vi "ConfigureFPGATach.vi"(8 "error in (no error)":errorcluster, 9 "delay comp":u32, 10 "keyphasor config":T1[](array[typedef]), 11 "dynamic FPGA VI reference":refnum<k20>) -> (0 "error out":errorcluster, 3 "dynamic FPGA VI reference":refnum<k20>)   [LabVIEW 2017, in "cRIOWfmLib.lvlib"]
uses:
  <vilib>/addons/InsightCM/Devices/Shared/Cms/cRIOWfmAcq/cRIOWfmLib.lvlib
  <vilib>/addons/InsightCM/Devices/Shared/Cms/CmsAcquisition/controls/TachometerConfig.ctl
  <vilib>/Utility/error.llb/Error Cluster From Error Code.vi
  <vilib>/rvi/errors/niLvFpgaAdjustHostInterfaceError.vi
  <vilib>/rvi/interface/nirviReadWriteControl/nirviReadWriteControl.xnode
  NiFpgaLv.dll
  <vilib>/rvi/interface/Simulation/niFpgaSimulationCallBeginRW.vi
  <vilib>/addons/InsightCM/Devices/Shared/Cms/CmsAcquisition/CmsAcquisition.lvlib
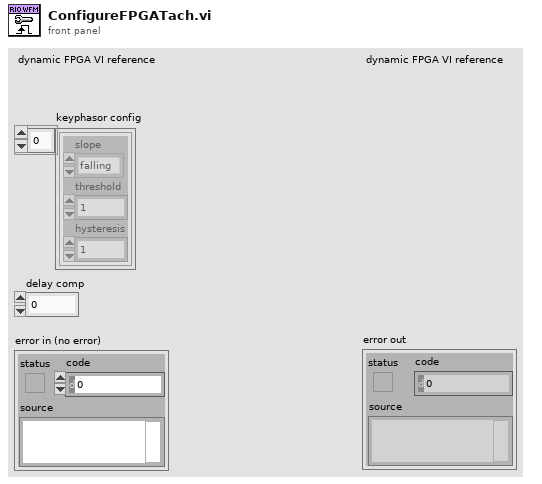
[diagram p1: front panel]
types:
  T1 = typedef "CmsAcquisition.lvlib/TachometerConfig.ctl" = cluster{"slope":enum16{"falling", "rising"}, "threshold":dbl, "hysteresis":dbl}
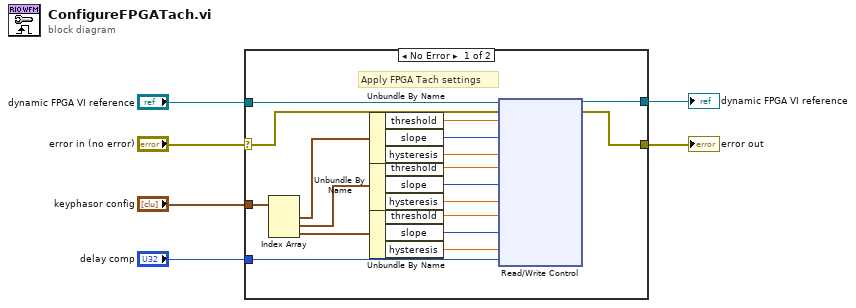
[diagram p0: block diagram]
diagram:
  n1 = case shown="No Error" "error in (no error)" {
    selector: "error in (no error)" -> [w23 w25]
    tunnel: "dynamic FPGA VI reference" -> [w24 w26]
    tunnel: [w22 w26] -> w1
    tunnel: [w21 w25] -> w5
    tunnel: "delay comp" -> [w20 _]
    tunnel: "keyphasor config" -> [w19 _]
    frame No Error {
      # "Apply FPGA Tach settings"
      n2 = Index Array(array=w19) -> (element #1=w18:T1, element #2=w8:T1, element #3=w7:T1)  [unwired: 3 in]
      n3 = Unbundle By Name(w18) -> ("threshold"=w17:dbl, "slope"=w16:enum16{"falling", "rising"}, "hysteresis"=w15:dbl)
      n4 = Unbundle By Name(w8) -> ("threshold"=w14:dbl, "slope"=w13:enum16{"falling", "rising"}, "hysteresis"=w12:dbl)
      n5 = Unbundle By Name(w7) -> ("threshold"=w11:dbl, "slope"=w10:enum16{"falling", "rising"}, "hysteresis"=w9:dbl)
      n6 = xnode "Read/Write Control"("FPGA VI Reference In"=w24, "error in"=w23, "Threshold0"=w17, "Slope0"=w16, "Hysteresis0"=w15, "Threshold1"=w14, "Slope1"=w13, "Hysteresis1"=w12, "Threshold2"=w11, "Slope2"=w10, "Hysteresis2"=w9, "Delay Comp"=w20) -> ("FPGA VI Reference Out"=w22:refnum<k20>, "error out"=w21:errorcluster)
    }
    frame Error {
    }
  }
  "error out" <- w5
  "dynamic FPGA VI reference" <- w1
